vi "swerve_best_angle.vi"(6 "Current Angle":dbl format="%#_13g", 7 "Target Angle":dbl format="%#_13g", 8 "Power In":dbl) -> (0 "Setpoint Angle":dbl format="%_4g", 3 "Power Out":dbl)   [LabVIEW 2020]
doc: "Based on the Current Angle and the Goal Angle, this VI calulates the signed angular distance. Taking into account the option to invert the direction of the swerve drive motor and always picking the shortest travel distance. The hysteresis prevents undesirable vacillation between angle choices."
uses:
  <vilib>/Analysis/coordinate.llb/Angle Range (Degree).ctl
  <vilib>/Analysis/coordinate.llb/Angle Units.ctl
  <vilib>/Analysis/coordinate.llb/Wrap Angle (scalar).vi
  <vilib>/Analysis/NI_AAL_Angle.lvlib
panel:
  # "(deg) [-180,+180]"
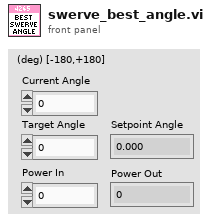
[diagram p1: front panel]
types:
  T1 = typedef "NI_AAL_Angle.lvlib/Angle Range (Degree).ctl" = u16
  T2 = typedef "NI_AAL_Angle.lvlib/Angle Units.ctl" = i32
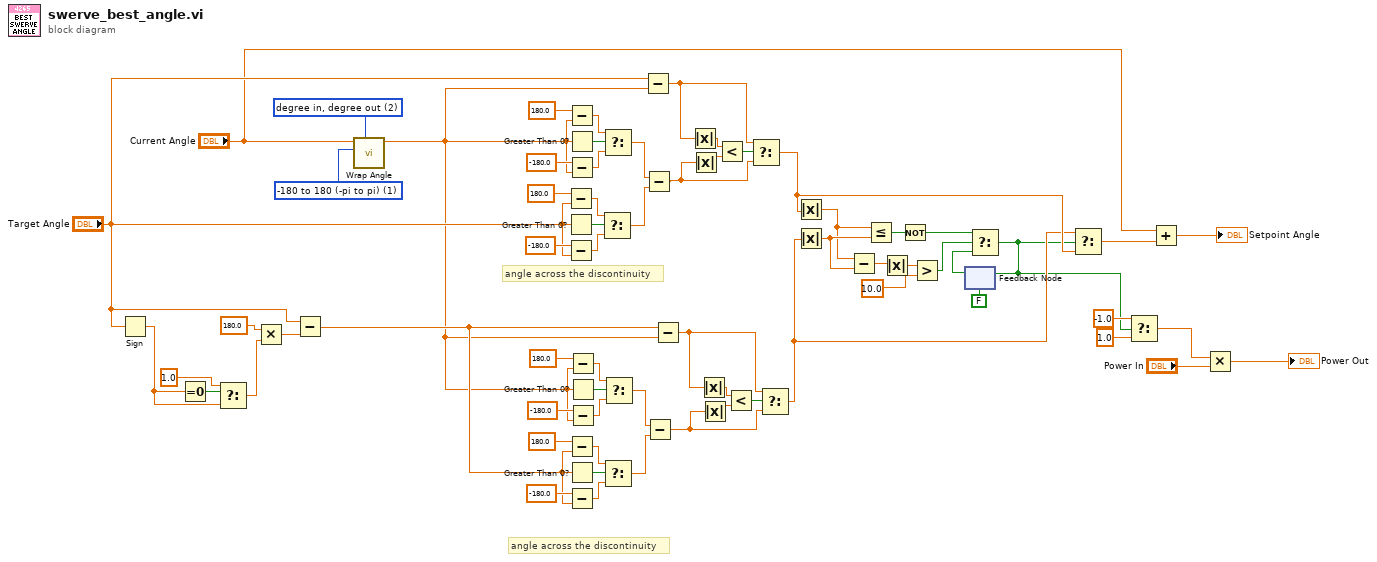
[diagram p0: block diagram]
diagram:
  w5 = T1 1 items=["none", "-180 to 180 (-pi to pi)", "0 to 360 (0 to 2pi)"] ("angle range")
  w6 = T2 2 items=["radian in, radian out", "radian in, degree out", "degree in, degree out", "degree in, radian out"] ("angle units")
  # "angle across the discontinuity"
  # "angle across the discontinuity"
  n1 = Sign(1:"Target Angle") -> (0:w20:dbl)
  n2 = Equal To 0?(x=w20) -> (x = 0?=w21:bool)
  n3 = Select(t=1.0, s=w21, f=w20) -> (s? t:f=w17:dbl)
  n4 = Multiply(x=180.0 ("y"), y=w17) -> (x*y=w66:dbl)
  n5 = Subtract(x="Target Angle", y=w66) -> (x-y=w41:dbl)
  n6 = call-poly <vilib>:"Wrap Angle.vi"("angle units"=w6, "angle range"=w5, "angle in"="Current Angle") -> ("angle out"=w2:dbl)  [unwired: 7 in, 1 out]
  n7 = Subtract(x=180.0, y="Target Angle") -> (x-y=w29:dbl)
  n8 = Greater Than 0?(x="Target Angle") -> (x > 0?=w31:bool)
  n9 = Subtract(x=-180.0, y="Target Angle") -> (x-y=w27:dbl)
  n10 = Subtract(x=180.0, y=w2) -> (x-y=w34:dbl)
  n11 = Greater Than 0?(x=w2) -> (x > 0?=w36:bool)
  n12 = Subtract(x=-180.0, y=w2) -> (x-y=w32:dbl)
  n13 = Subtract(x=180.0, y=w41) -> (x-y=w50:dbl)
  n14 = Greater Than 0?(x=w41) -> (x > 0?=w52:bool)
  n15 = Subtract(x=-180.0, y=w41) -> (x-y=w48:dbl)
  n16 = Subtract(x=180.0, y=w2) -> (x-y=w56:dbl)
  n17 = Greater Than 0?(x=w2) -> (x > 0?=w58:bool)
  n18 = Subtract(x=-180.0, y=w2) -> (x-y=w54:dbl)
  n19 = Select(t=w29, s=w31, f=w27) -> (s? t:f=w25:dbl)
  n20 = Select(t=w34, s=w36, f=w32) -> (s? t:f=w26:dbl)
  n21 = Select(t=w50, s=w52, f=w48) -> (s? t:f=w46:dbl)
  n22 = Select(t=w56, s=w58, f=w54) -> (s? t:f=w47:dbl)
  n23 = Subtract(x="Target Angle", y=w2) -> (x-y=w37:dbl)
  n24 = Subtract(x=w26, y=w25) -> (x-y=w24:dbl)
  n25 = Subtract(x=w47, y=w46) -> (x-y=w45:dbl)
  n26 = Subtract(x=w41, y=w2) -> (x-y=w42:dbl)
  n27 = Absolute Value(x=w37) -> (abs(x)=w38:dbl)
  n28 = Absolute Value(x=w24) -> (abs(x)=w39:dbl)
  n29 = Absolute Value(x=w42) -> (abs(x)=w43:dbl)
  n30 = Absolute Value(x=w45) -> (abs(x)=w44:dbl)
  n31 = Less?(x=w38, y=w39) -> (x < y?=w40:bool)
  n32 = Less?(x=w43, y=w44) -> (x < y?=w53:bool)
  n33 = Select(t=w37, s=w40, f=w24) -> (s? t:f=w16:dbl)
  n34 = Select(t=w42, s=w53, f=w45) -> (s? t:f=w15:dbl)
  n35 = Absolute Value(x=w16) -> (abs(x)=w59:dbl)
  n36 = Absolute Value(x=w15) -> (abs(x)=w60:dbl)
  n37 = Subtract(x=w59, y=w60) -> (x-y=w63:dbl)
  n38 = Less Or Equal?(x=w59, y=w60) -> (x <= y?=w23:bool)
  n39 = Absolute Value(x=w63) -> (abs(x)=w62:dbl)
  n40 = Not(x=w23) -> (.not. x?=w22:bool)
  n41 = Greater?(x=w62, y=10.0) -> (0:w61:bool)
  n42 = feedback #1(FALSE) -> (w65:bool)
  n43 = Select(t=w22, s=w61, f=w65) -> (s? t:f=w7:bool)
  n44 = feedback-in #1(w7) -> ()
  n45 = Select(t=w15, s=w7, f=w16) -> (s? t:f=w4:dbl)
  n46 = Select(t=-1.0, s=w7, f=1.0) -> (s? t:f=w12:dbl)
  n47 = Add(x="Current Angle", y=w4) -> (x+y=→"Setpoint Angle":dbl)
  n48 = Multiply(x=w12, y="Power In") -> (x*y=→"Power Out":dbl)
